vi "Example_Set_Get Functios.vi"() -> ()   [LabVIEW 2020]
doc: "Demonstrates the most used functions of the VI Server Toolkit - getting or setting control values based on two polymorphic VIs."
uses:
  VI Server Toolkit LV2013.lvlib
  VI Server Libraries/VI Server_Set Controls.llb/Set DBL SLIDE Control.vi
  VI Server Libraries/VI Server_Set Controls.llb/Set DBL Knob Control.vi
  VI Server Libraries/VI Server_Set Controls.llb/Set 1D STR Control.vi
  VI Server Libraries/VI Server_Set Controls.llb/Set STR Control.vi
panel:
  in  "Tab.Main":enum32{"Set/Get1", "Set/Get2"}(tab)
  in  "Menu Ring.Item Names":string[](array[string])=["Item 1", "Item 2", "Item 3"] caption="1D Array - String"
  in  "Slide.Get":bool
  in  "Slide.Set":bool
  in  "Menu Ring.Get":bool
  in  "Menu Ring.Set":bool
  in  "File Path.Source":path
  in  "Numeric.Source":dbl=5.0 caption="Numeric Control"
  in  "Slide.Source":dbl(slide)=1.9191919191919191 caption="Horizontal Fill Slide" scale=0.0..10.0
  in  "Knob.Source":dbl(knob)=1.6969989516945825 caption="Knob" scale=0.0..10.0
  in  "Button.Source":bool caption="Settings Button"
  in  "Menu Ring.Source":u16(ring) caption="Menu Ring" items=["Item 1", "Item 2", "Item 3"]
  in  "LED.Source":bool caption="LED"
  in  "File Path.Get":bool
  in  "File Path.Set":bool
  in  "LED.Get":bool
  in  "LED.Set":bool
  in  "Button.Get":bool
  in  "Button.Set":bool
  in  "Knob.Get":bool
  in  "Knob.Set":bool
  in  "Numeric.Get":bool
  in  "Numeric.Set":bool
  in  "File Path.Mirror":path
  in  "Numeric.Mirror":dbl=5.0 caption="Numeric Control"
  in  "Slide.Mirror":dbl(slide)=1.9191919191919191 caption="Horizontal Fill Slide" scale=0.0..10.0
  in  "Knob.Mirror":dbl(knob) caption="Knob" scale=0.0..10.0
  in  "Button.Mirror":bool caption="Settings Button"
  in  "Menu Ring.Mirror":u16(ring) caption="Menu Ring" items=["Item 1", "Item 2", "Item 3"]
  in  "LED.Mirror":bool caption="LED"
  in  "2D Array - Path.Get":bool
  in  "2D Array - Path.Set":bool
  in  "2D Array - DBL.Get":bool
  in  "2D Array - DBL.Set":bool
  in  "1D Array - DBL.Get":bool
  in  "1D Array - DBL.Set":bool
  in  "2D Array - String.Get":bool
  in  "2D Array - String.Set":bool
  in  "1D Array - String.Mirror":string[](array[string]) caption="1D Array - String"
  in  "2D Array - String.Mirror":string[][](array[string]) caption="2D Array - String"
  in  "1D Array - DBL.Mirror":dbl[](array[numeric]) caption="1D Array - DBL"
  in  "2D Array - DBL.Mirror":dbl[][](array[numeric]) caption="2D Array - DBL"
  in  "2D Array - Path.Mirror":path[][](array[path]) caption="2D Array - String"
  in  "2D Array - Boolean.Mirror":bool[][](array[boolean]) caption="2D Array - String"
  in  "1D Array - String.Source":string[](array[string]) caption="1D Array - String"
  in  "2D Array - String.Source":string[][](array[string])=[["", ""], ["", ""], ["", "qwe"]] caption="2D Array - String"
  in  "1D Array - DBL.Source":dbl[](array[numeric]) caption="1D Array - DBL"
  in  "2D Array - DBL.Source":dbl[][](array[numeric]) caption="2D Array - DBL"
  in  "2D Array - Path.Source":path[][](array[path]) caption="2D Array - String"
  in  "2D Array - Boolean.Source":bool[][](array[boolean]) caption="2D Array - String"
  in  "1D Array - String.Get":bool
  in  "1D Array - String.Set":bool
  in  "2D Array - Path.Get":bool
  in  "2D Array - Path.Set":bool
  in  "EXIT":bool=TRUE
  in  "Error In":errorcluster
  out "error out":errorcluster
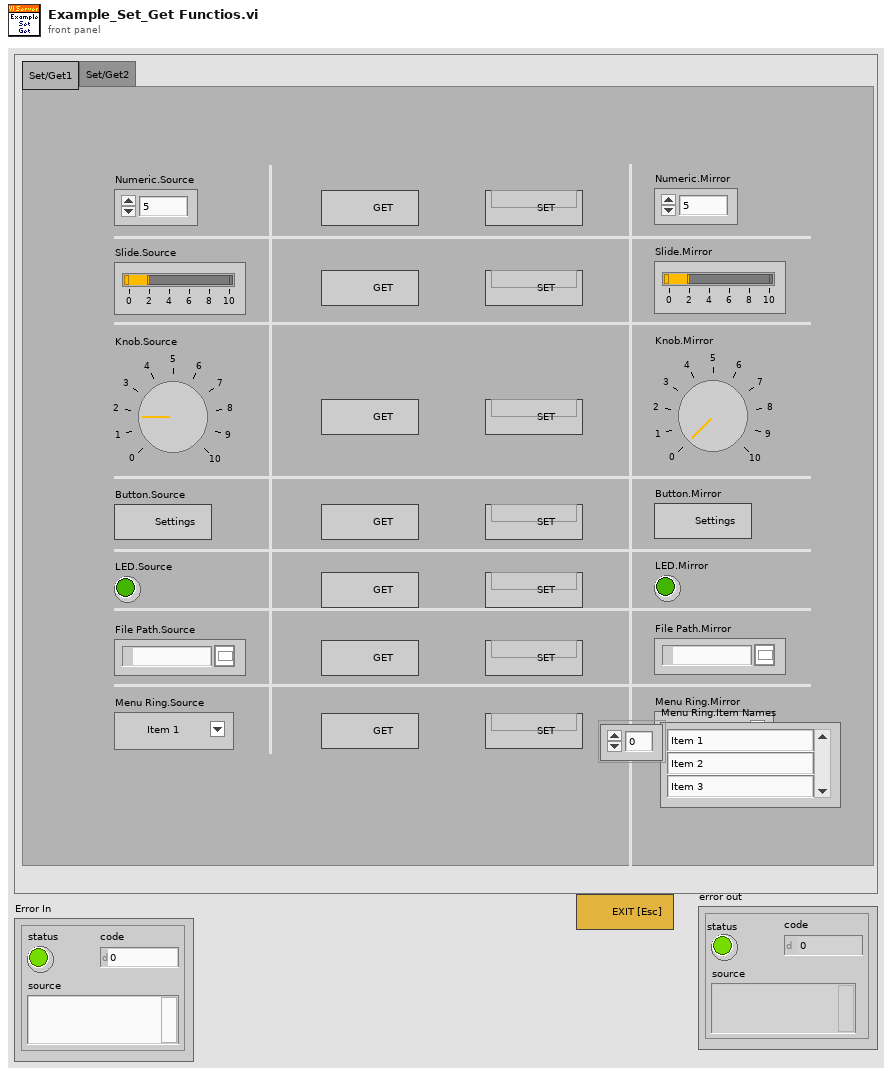
[diagram p1: front panel]
types:
  T1 = typedef "VI Server_RefsCluster.ctl" = cluster{"Labels":string[], "Refs":refnum<vi>[], "VI Ref":refnum<vi>}
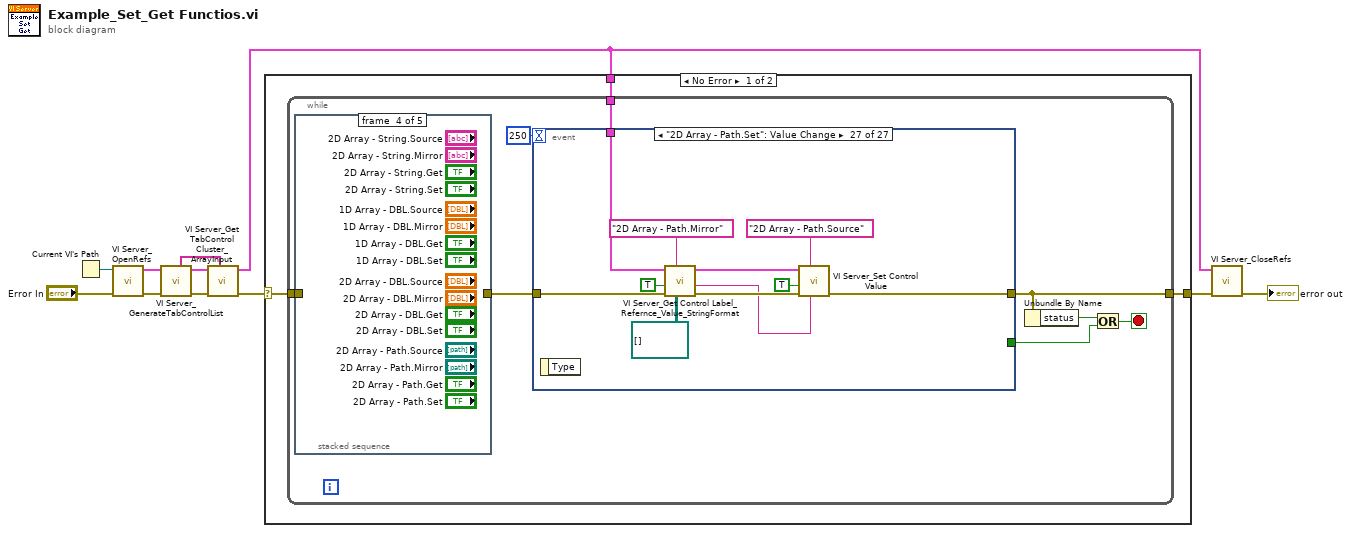
[diagram p0: block diagram]
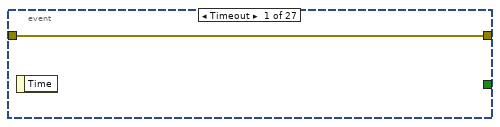
[diagram p2: hidden frame]
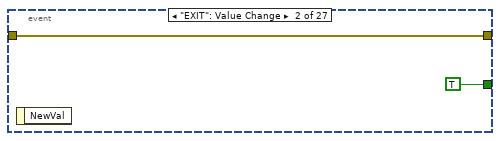
[diagram p3: hidden frame]
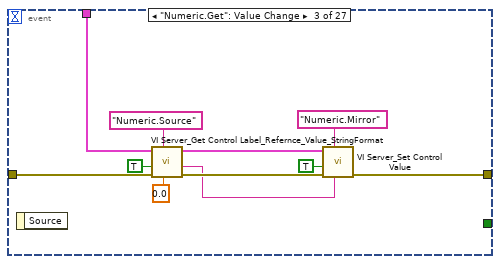
[diagram p4: hidden frame]
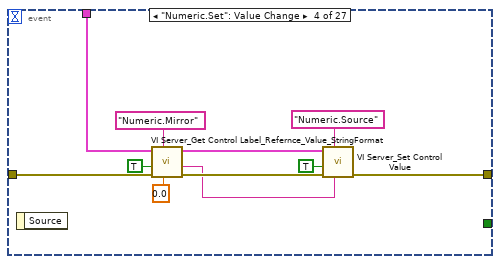
[diagram p5: hidden frame]
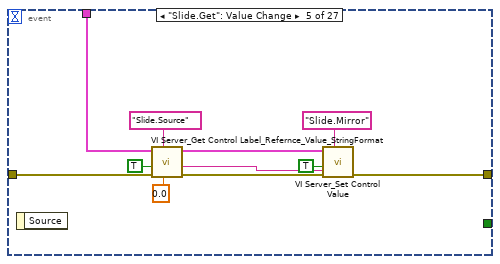
[diagram p6: hidden frame]
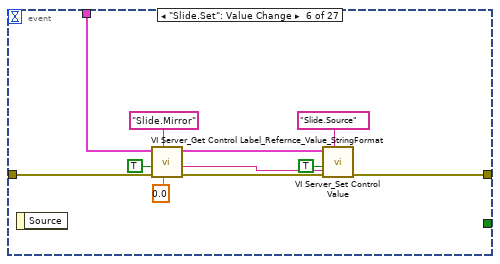
[diagram p7: hidden frame]
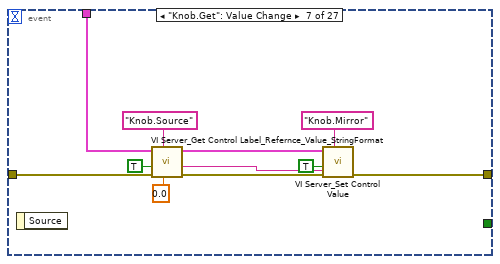
[diagram p8: hidden frame]
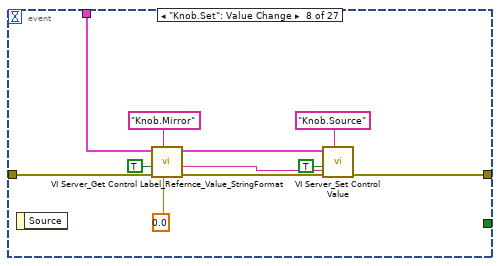
[diagram p9: hidden frame]
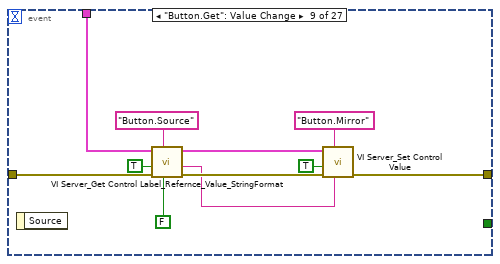
[diagram p10: hidden frame]
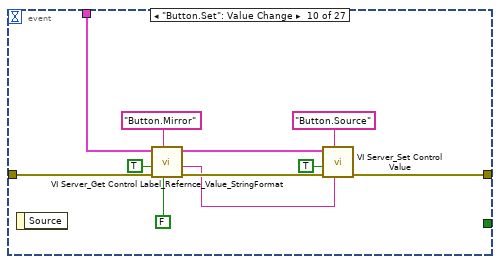
[diagram p11: hidden frame]
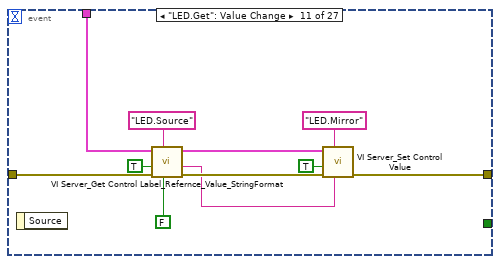
[diagram p12: hidden frame]
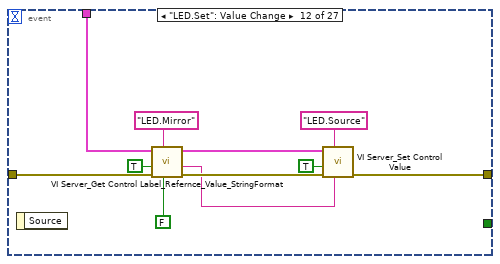
[diagram p13: hidden frame]
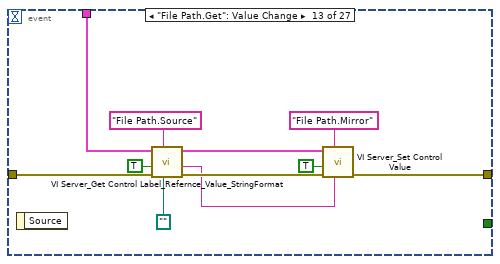
[diagram p14: hidden frame]
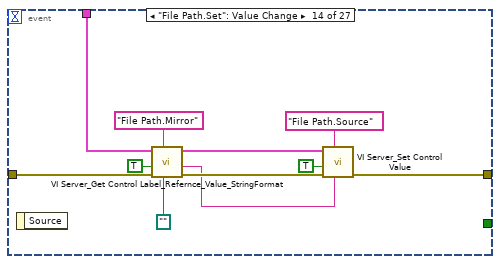
[diagram p15: hidden frame]
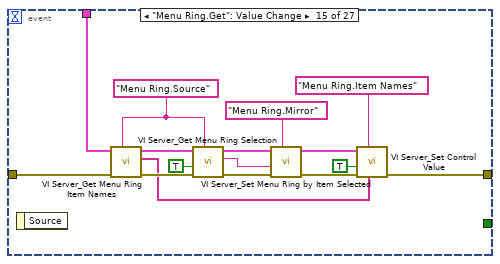
[diagram p16: hidden frame]
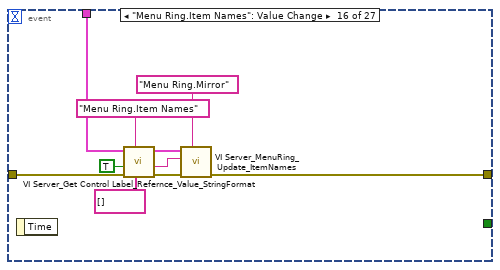
[diagram p17: hidden frame]
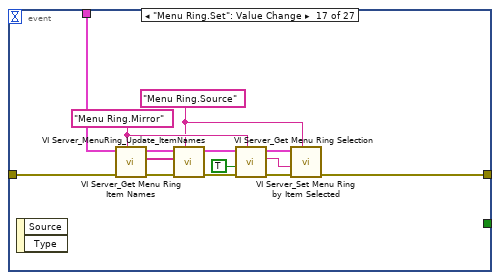
[diagram p18: hidden frame]
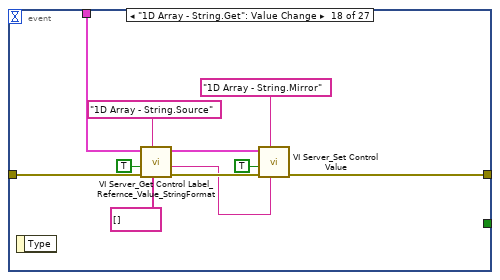
[diagram p19: hidden frame]
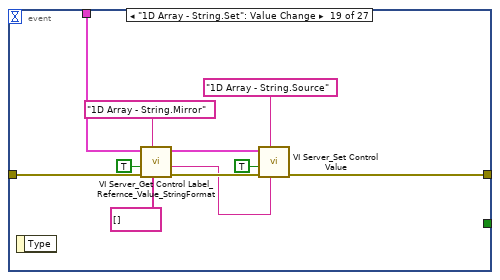
[diagram p20: hidden frame]
diagram:
  n1 = Current VI's Path() -> (path=w10:path)
  n2 = call "VI Server_OpenRefs.vi"("error in"="Error In", "VI Path"=w10) -> ("error out"=w4:errorcluster, "VI Server.RefsCluster"=w5:T1)  [unwired: 8 in]
  n3 = call "VI Server_GenerateTabControlList.vi"("error in (no error)"=w4, "VI Server Cluster"=w5) -> ("error out"=w7:errorcluster, "VI Server Cluster.DUP"=w6:T1, "TabControls"=w2:string[])  [unwired: 7 in]
  n4 = call "VI Server_Get TabControl Cluster_ArrayInput.vi"("TabControl Labels[]"=w2, "error in"=w7, "VI Server Cluster"=w6) -> ("error out"=w3:errorcluster, "VI Server Cluster.OUT"=w1:T1)  [unwired: 7 in]
  n5 = case shown="No Error" w3 {
    selector: w3 -> [w14 w309]
    tunnel: [w13 w309] -> w9
    tunnel: w1 -> [w12 _]
    frame No Error {
      n6 = while {
        tunnel: w14 -> [w21]
        tunnel: [w19] -> w13
        tunnel: w12 -> [w15]
        stop <- w16 stop-if-true
        n7 = stacked-sequence {
          tunnel: [w308 _ _ _ _] -> w20
          tunnel: w21 -> [w308 _ _ _ _]
          frame #0 {
          }
          frame #1 {
          }
          frame #2 {
          }
          frame #3 {
          }
          frame #4 {
          }
        }
        n8 = event shown="[26] \"2D Array - Path.Set\": Value Change" {
          selector: _ -> [_ _ _ _ _ _ _ _ _ _ _ _ _ _ _ _ _ _ _ _ _ _ _ _ _ _ _]
          dyn-events: _ -> [_ _ _ _ _ _ _ _ _ _ _ _ _ _ _ _ _ _ _ _ _ _ _ _ _ _ _]
          timeout: 250 -> [_ _ _ _ _ _ _ _ _ _ _ _ _ _ _ _ _ _ _ _ _ _ _ _ _ _ _]
          tunnel: w20 -> [w23 w25 w36 w47 w58 w69 w80 w91 w102 w113 w124 w135 w146 w157 w165 w183 w197 w208 w219 w230 w241 w252 w263 w274 w285 w296 w307]
          tunnel: [w23 w25 w30 w41 w52 w63 w74 w85 w96 w107 w118 w129 w140 w151 w159 w174 w186 w200 w211 w222 w233 w244 w255 w266 w277 w288 w299] -> w19
          tunnel: [_ TRUE _ _ _ _ _ _ _ _ _ _ _ _ _ _ _ _ _ _ _ _ _ _ _ _ _] -> w17
          tunnel: w15 -> [_ _ w35 w46 w57 w68 w79 w90 w101 w112 w123 w134 w145 w156 w163 w182 w196 w207 w218 w229 w240 w251 w262 w273 w284 w295 w306]
          event Timeout {
            n9 = event-data() -> ()  [unwired: 1 in, 1 out]
          }
          event "EXIT": Value Change {
            n10 = event-data() -> ()  [unwired: 1 in, 1 out]
          }
          event "Numeric.Get": Value Change {
            n11 = event-data() -> ()  [unwired: 1 in, 1 out]
            n12 = call "VI Server_Get Control Label_Refernce_Value_StringFormat.vi"(6:0.0, "Label"="Numeric.Source", "error in (no error)"=w36, 9:TRUE ("Single Instance (T)"), "VI Server Cluster"=w35) -> ("error out"=w31:errorcluster, "ControlValue(StringFormat)"=w27:string, "VI Server Cluster.DUP"=w28:T1)  [unwired: 4 in]
            n13 = call-poly "VI Server_Set Control Value.vi"("New Value"=w27, "Label"="Numeric.Mirror", "error in"=w31, "Single Instance (T)"=TRUE, "VI Server Cluster"=w28) -> ("error out"=w30:errorcluster)  [unwired: 4 in, 2 out]
          }
          event "Numeric.Set": Value Change {
            n14 = event-data() -> ()  [unwired: 1 in, 1 out]
            n15 = call "VI Server_Get Control Label_Refernce_Value_StringFormat.vi"(6:0.0, "Label"="Numeric.Mirror", "error in (no error)"=w47, 9:TRUE ("Single Instance (T)"), "VI Server Cluster"=w46) -> ("error out"=w42:errorcluster, "ControlValue(StringFormat)"=w38:string, "VI Server Cluster.DUP"=w39:T1)  [unwired: 4 in]
            n16 = call-poly "VI Server_Set Control Value.vi"("New Value"=w38, "Label"="Numeric.Source", "error in"=w42, "Single Instance (T)"=TRUE, "VI Server Cluster"=w39) -> ("error out"=w41:errorcluster)  [unwired: 4 in, 2 out]
          }
          event "Slide.Get": Value Change {
            n17 = event-data() -> ()  [unwired: 1 in, 1 out]
            n18 = call "VI Server_Get Control Label_Refernce_Value_StringFormat.vi"(6:0.0, "Label"="Slide.Source", "error in (no error)"=w58, 9:TRUE ("Single Instance (T)"), "VI Server Cluster"=w57) -> ("error out"=w53:errorcluster, "ControlValue(StringFormat)"=w49:string, "VI Server Cluster.DUP"=w50:T1)  [unwired: 4 in]
            n19 = call-poly "VI Server_Set Control Value.vi"("New Value"=w49, "Label"="Slide.Mirror", "error in"=w53, "Single Instance (T)"=TRUE, "VI Server Cluster"=w50) -> ("error out"=w52:errorcluster)  [unwired: 4 in, 2 out]
          }
          event "Slide.Set": Value Change {
            n20 = event-data() -> ()  [unwired: 1 in, 1 out]
            n21 = call "VI Server_Get Control Label_Refernce_Value_StringFormat.vi"(6:0.0, "Label"="Slide.Mirror", "error in (no error)"=w69, 9:TRUE ("Single Instance (T)"), "VI Server Cluster"=w68) -> ("error out"=w64:errorcluster, "ControlValue(StringFormat)"=w60:string, "VI Server Cluster.DUP"=w61:T1)  [unwired: 4 in]
            n22 = call-poly "VI Server_Set Control Value.vi"("New Value"=w60, "Label"="Slide.Source", "error in"=w64, "Single Instance (T)"=TRUE, "VI Server Cluster"=w61) -> ("error out"=w63:errorcluster)  [unwired: 4 in, 2 out]
          }
          event "Knob.Get": Value Change {
            n23 = event-data() -> ()  [unwired: 1 in, 1 out]
            n24 = call "VI Server_Get Control Label_Refernce_Value_StringFormat.vi"(6:0.0, "Label"="Knob.Source", "error in (no error)"=w80, 9:TRUE ("Single Instance (T)"), "VI Server Cluster"=w79) -> ("error out"=w75:errorcluster, "ControlValue(StringFormat)"=w71:string, "VI Server Cluster.DUP"=w72:T1)  [unwired: 4 in]
            n25 = call-poly "VI Server_Set Control Value.vi"("New Value"=w71, "Label"="Knob.Mirror", "error in"=w75, "Single Instance (T)"=TRUE, "VI Server Cluster"=w72) -> ("error out"=w74:errorcluster)  [unwired: 4 in, 2 out]
          }
          event "Knob.Set": Value Change {
            n26 = event-data() -> ()  [unwired: 1 in, 1 out]
            n27 = call "VI Server_Get Control Label_Refernce_Value_StringFormat.vi"(6:0.0, "Label"="Knob.Mirror", "error in (no error)"=w91, 9:TRUE ("Single Instance (T)"), "VI Server Cluster"=w90) -> ("error out"=w86:errorcluster, "ControlValue(StringFormat)"=w82:string, "VI Server Cluster.DUP"=w83:T1)  [unwired: 4 in]
            n28 = call-poly "VI Server_Set Control Value.vi"("New Value"=w82, "Label"="Knob.Source", "error in"=w86, "Single Instance (T)"=TRUE, "VI Server Cluster"=w83) -> ("error out"=w85:errorcluster)  [unwired: 4 in, 2 out]
          }
          event "Button.Get": Value Change {
            n29 = event-data() -> ()  [unwired: 1 in, 1 out]
            n30 = call "VI Server_Get Control Label_Refernce_Value_StringFormat.vi"(6:FALSE, "Label"="Button.Source", "error in (no error)"=w102, 9:TRUE ("Single Instance (T)"), "VI Server Cluster"=w101) -> ("error out"=w97:errorcluster, "ControlValue(StringFormat)"=w93:string, "VI Server Cluster.DUP"=w94:T1)  [unwired: 4 in]
            n31 = call-poly "VI Server_Set Control Value.vi"("New Value"=w93, "Label"="Button.Mirror", "error in"=w97, "Single Instance (T)"=TRUE, "VI Server Cluster"=w94) -> ("error out"=w96:errorcluster)  [unwired: 4 in, 2 out]
          }
          event "Button.Set": Value Change {
            n32 = event-data() -> ()  [unwired: 1 in, 1 out]
            n33 = call "VI Server_Get Control Label_Refernce_Value_StringFormat.vi"(6:FALSE, "Label"="Button.Mirror", "error in (no error)"=w113, 9:TRUE ("Single Instance (T)"), "VI Server Cluster"=w112) -> ("error out"=w108:errorcluster, "ControlValue(StringFormat)"=w104:string, "VI Server Cluster.DUP"=w105:T1)  [unwired: 4 in]
            n34 = call-poly "VI Server_Set Control Value.vi"("New Value"=w104, "Label"="Button.Source", "error in"=w108, "Single Instance (T)"=TRUE, "VI Server Cluster"=w105) -> ("error out"=w107:errorcluster)  [unwired: 4 in, 2 out]
          }
          event "LED.Get": Value Change {
            n35 = event-data() -> ()  [unwired: 1 in, 1 out]
            n36 = call "VI Server_Get Control Label_Refernce_Value_StringFormat.vi"(6:FALSE, "Label"="LED.Source", "error in (no error)"=w124, 9:TRUE ("Single Instance (T)"), "VI Server Cluster"=w123) -> ("error out"=w119:errorcluster, "ControlValue(StringFormat)"=w115:string, "VI Server Cluster.DUP"=w116:T1)  [unwired: 4 in]
            n37 = call-poly "VI Server_Set Control Value.vi"("New Value"=w115, "Label"="LED.Mirror", "error in"=w119, "Single Instance (T)"=TRUE, "VI Server Cluster"=w116) -> ("error out"=w118:errorcluster)  [unwired: 4 in, 2 out]
          }
          event "LED.Set": Value Change {
            n38 = event-data() -> ()  [unwired: 1 in, 1 out]
            n39 = call "VI Server_Get Control Label_Refernce_Value_StringFormat.vi"(6:FALSE, "Label"="LED.Mirror", "error in (no error)"=w135, 9:TRUE ("Single Instance (T)"), "VI Server Cluster"=w134) -> ("error out"=w130:errorcluster, "ControlValue(StringFormat)"=w126:string, "VI Server Cluster.DUP"=w127:T1)  [unwired: 4 in]
            n40 = call-poly "VI Server_Set Control Value.vi"("New Value"=w126, "Label"="LED.Source", "error in"=w130, "Single Instance (T)"=TRUE, "VI Server Cluster"=w127) -> ("error out"=w129:errorcluster)  [unwired: 4 in, 2 out]
          }
          event "File Path.Get": Value Change {
            n41 = event-data() -> ()  [unwired: 1 in, 1 out]
            n42 = call "VI Server_Get Control Label_Refernce_Value_StringFormat.vi"(6:path "", "Label"="File Path.Source", "error in (no error)"=w146, 9:TRUE ("Single Instance (T)"), "VI Server Cluster"=w145) -> ("error out"=w141:errorcluster, "ControlValue(StringFormat)"=w137:string, "VI Server Cluster.DUP"=w138:T1)  [unwired: 4 in]
            n43 = call-poly "VI Server_Set Control Value.vi"("New Value"=w137, "Label"="File Path.Mirror", "error in"=w141, "Single Instance (T)"=TRUE, "VI Server Cluster"=w138) -> ("error out"=w140:errorcluster)  [unwired: 4 in, 2 out]
          }
          event "File Path.Set": Value Change {
            n44 = event-data() -> ()  [unwired: 1 in, 1 out]
            n45 = call "VI Server_Get Control Label_Refernce_Value_StringFormat.vi"(6:path "", "Label"="File Path.Mirror", "error in (no error)"=w157, 9:TRUE ("Single Instance (T)"), "VI Server Cluster"=w156) -> ("error out"=w152:errorcluster, "ControlValue(StringFormat)"=w148:string, "VI Server Cluster.DUP"=w149:T1)  [unwired: 4 in]
            n46 = call-poly "VI Server_Set Control Value.vi"("New Value"=w148, "Label"="File Path.Source", "error in"=w152, "Single Instance (T)"=TRUE, "VI Server Cluster"=w149) -> ("error out"=w151:errorcluster)  [unwired: 4 in, 2 out]
          }
          event "Menu Ring.Get": Value Change {
            w161 = "Menu Ring.Source" ("Label")
            n47 = event-data() -> ()  [unwired: 1 in, 1 out]
            n48 = call "VI Server_Get Menu Ring Item Names.vi"("Label"=w161, "error in"=w165, "VI Server Cluster"=w163) -> ("error out"=w164:errorcluster, "Item Names (String[])"=w160:string[], "VI Server Cluster.DUP"=w162:T1)  [unwired: 3 in, 3 out]
            n49 = call "VI Server_Get Menu Ring Selection.vi"("Label"=w161, "error in"=w164, "Single Instance (T)"=TRUE, "VI Server Cluster"=w162) -> ("error out"=w172:errorcluster, "Selection"=w170:string, "VI Server Cluster.DUP"=w167:T1)  [unwired: 2 in, 3 out]
            n50 = call "VI Server_Set Menu Ring by Item Selected.vi"("Label"="Menu Ring.Mirror", "error in"=w172, "Item"=w170, "VI Server Cluster"=w167) -> ("error out"=w169:errorcluster, "VI Server Cluster.DUP"=w168:T1)  [unwired: 5 in, 1 out]
            n51 = call-poly "VI Server_Set Control Value.vi"("New Value"=w160, "Label"="Menu Ring.Item Names", "error in"=w169, "Single Instance (T)"=TRUE, "VI Server Cluster"=w168) -> ("error out"=w159:errorcluster)  [unwired: 4 in, 2 out]
          }
          event "Menu Ring.Item Names": Value Change {
            n52 = event-data() -> ()  [unwired: 1 in, 1 out]
            n53 = call "VI Server_Get Control Label_Refernce_Value_StringFormat.vi"(6:string[] [], "Label"="Menu Ring.Item Names", "error in (no error)"=w183, 9:TRUE ("Single Instance (T)"), "VI Server Cluster"=w182) -> ("error out"=w178:errorcluster, "ControlValue(StringFormat)"=w175:string, "VI Server Cluster.DUP"=w177:T1)  [unwired: 4 in]
            n54 = call "VI Server_MenuRing_Update_ItemNames.vi"("Label"="Menu Ring.Mirror", "error in"=w178, "Strings []"=w175, "VI Server Cluster"=w177) -> ("error out"=w174:errorcluster)  [unwired: 5 in, 2 out]
          }
          event "Menu Ring.Set": Value Change {
            w185 = "Menu Ring.Source"
            w191 = "Menu Ring.Mirror"
            n55 = event-data() -> ()  [unwired: 1 in, 2 out]
            n56 = call "VI Server_Get Menu Ring Item Names.vi"("Label"=w191, "error in"=w197, "VI Server Cluster"=w196) -> ("error out"=w195:errorcluster, "Item Names (String[])"=w193:string[], "VI Server Cluster.DUP"=w194:T1)  [unwired: 3 in, 3 out]
            n57 = call "VI Server_MenuRing_Update_ItemNames.vi"("Label"=w185, "error in"=w195, "Strings []"=w193, "VI Server Cluster"=w194) -> ("error out"=w192:errorcluster, "VI Server Cluster.DUP"=w190:T1)  [unwired: 5 in, 1 out]
            n58 = call "VI Server_Get Menu Ring Selection.vi"("Label"=w191, "error in"=w192, "Single Instance (T)"=TRUE, "VI Server Cluster"=w190) -> ("error out"=w188:errorcluster, "Selection"=w184:string, "VI Server Cluster.DUP"=w187:T1)  [unwired: 2 in, 3 out]
            n59 = call "VI Server_Set Menu Ring by Item Selected.vi"("Label"=w185, "error in"=w188, "Item"=w184, "VI Server Cluster"=w187) -> ("error out"=w186:errorcluster)  [unwired: 5 in, 2 out]
          }
          event "1D Array - String.Get": Value Change {
            n60 = event-data() -> ()  [unwired: 1 in, 1 out]
            n61 = call "VI Server_Get Control Label_Refernce_Value_StringFormat.vi"(6:string[] [], "Label"="1D Array - String.Source", "error in (no error)"=w208, 9:TRUE ("Single Instance (T)"), "VI Server Cluster"=w207) -> ("error out"=w203:errorcluster, "ControlValue(StringFormat)"=w198:string, "VI Server Cluster.DUP"=w202:T1)  [unwired: 4 in]
            n62 = call-poly "VI Server_Set Control Value.vi"("New Value"=w198, "Label"="1D Array - String.Mirror", "error in"=w203, "Single Instance (T)"=TRUE, "VI Server Cluster"=w202) -> ("error out"=w200:errorcluster)  [unwired: 4 in, 2 out]
          }
          event "1D Array - String.Set": Value Change {
            n63 = event-data() -> ()  [unwired: 1 in, 1 out]
            n64 = call "VI Server_Get Control Label_Refernce_Value_StringFormat.vi"(6:string[] [], "Label"="1D Array - String.Mirror", "error in (no error)"=w219, 9:TRUE ("Single Instance (T)"), "VI Server Cluster"=w218) -> ("error out"=w214:errorcluster, "ControlValue(StringFormat)"=w209:string, "VI Server Cluster.DUP"=w213:T1)  [unwired: 4 in]
            n65 = call-poly "VI Server_Set Control Value.vi"("New Value"=w209, "Label"="1D Array - String.Source", "error in"=w214, "Single Instance (T)"=TRUE, "VI Server Cluster"=w213) -> ("error out"=w211:errorcluster)  [unwired: 4 in, 2 out]
          }
          event "2D Array - String.Get": Value Change {
            n66 = event-data() -> ()  [unwired: 1 in, 1 out]
            n67 = call "VI Server_Get Control Label_Refernce_Value_StringFormat.vi"(6:string[][] [], "Label"="2D Array - String.Source", "error in (no error)"=w230, 9:TRUE ("Single Instance (T)"), "VI Server Cluster"=w229) -> ("error out"=w225:errorcluster, "ControlValue(StringFormat)"=w220:string, "VI Server Cluster.DUP"=w224:T1)  [unwired: 4 in]
            n68 = call-poly "VI Server_Set Control Value.vi"("New Value"=w220, "Label"="2D Array - String.Mirror", "error in"=w225, "Single Instance (T)"=TRUE, "VI Server Cluster"=w224) -> ("error out"=w222:errorcluster)  [unwired: 4 in, 2 out]
          }
          event "2D Array - String.Set": Value Change {
            n69 = event-data() -> ()  [unwired: 1 in, 1 out]
            n70 = call "VI Server_Get Control Label_Refernce_Value_StringFormat.vi"(6:string[][] [], "Label"="2D Array - String.Mirror", "error in (no error)"=w241, 9:TRUE ("Single Instance (T)"), "VI Server Cluster"=w240) -> ("error out"=w236:errorcluster, "ControlValue(StringFormat)"=w231:string, "VI Server Cluster.DUP"=w235:T1)  [unwired: 4 in]
            n71 = call-poly "VI Server_Set Control Value.vi"("New Value"=w231, "Label"="2D Array - String.Source", "error in"=w236, "Single Instance (T)"=TRUE, "VI Server Cluster"=w235) -> ("error out"=w233:errorcluster)  [unwired: 4 in, 2 out]
          }
          event "1D Array - DBL.Get": Value Change {
            n72 = event-data() -> ()  [unwired: 1 in, 1 out]
            n73 = call "VI Server_Get Control Label_Refernce_Value_StringFormat.vi"(6:dbl[] [], "Label"="1D Array - DBL.Source", "error in (no error)"=w252, 9:TRUE ("Single Instance (T)"), "VI Server Cluster"=w251) -> ("error out"=w247:errorcluster, "ControlValue(StringFormat)"=w242:string, "VI Server Cluster.DUP"=w246:T1)  [unwired: 4 in]
            n74 = call-poly "VI Server_Set Control Value.vi"("New Value"=w242, "Label"="1D Array - DBL.Mirror", "error in"=w247, "Single Instance (T)"=TRUE, "VI Server Cluster"=w246) -> ("error out"=w244:errorcluster)  [unwired: 4 in, 2 out]
          }
          event "1D Array - DBL.Set": Value Change {
            n75 = event-data() -> ()  [unwired: 1 in, 1 out]
            n76 = call "VI Server_Get Control Label_Refernce_Value_StringFormat.vi"(6:dbl[] [], "Label"="1D Array - DBL.Mirror", "error in (no error)"=w263, 9:TRUE ("Single Instance (T)"), "VI Server Cluster"=w262) -> ("error out"=w258:errorcluster, "ControlValue(StringFormat)"=w253:string, "VI Server Cluster.DUP"=w257:T1)  [unwired: 4 in]
            n77 = call-poly "VI Server_Set Control Value.vi"("New Value"=w253, "Label"="1D Array - DBL.Source", "error in"=w258, "Single Instance (T)"=TRUE, "VI Server Cluster"=w257) -> ("error out"=w255:errorcluster)  [unwired: 4 in, 2 out]
          }
          event "2D Array - DBL.Get": Value Change {
            n78 = event-data() -> ()  [unwired: 1 in, 1 out]
            n79 = call "VI Server_Get Control Label_Refernce_Value_StringFormat.vi"(6:dbl[][] [], "Label"="2D Array - DBL.Source", "error in (no error)"=w274, 9:TRUE ("Single Instance (T)"), "VI Server Cluster"=w273) -> ("error out"=w269:errorcluster, "ControlValue(StringFormat)"=w264:string, "VI Server Cluster.DUP"=w268:T1)  [unwired: 4 in]
            n80 = call-poly "VI Server_Set Control Value.vi"("New Value"=w264, "Label"="2D Array - DBL.Mirror", "error in"=w269, "Single Instance (T)"=TRUE, "VI Server Cluster"=w268) -> ("error out"=w266:errorcluster)  [unwired: 4 in, 2 out]
          }
          event "2D Array - DBL.Set": Value Change {
            n81 = event-data() -> ()  [unwired: 1 in, 1 out]
            n82 = call "VI Server_Get Control Label_Refernce_Value_StringFormat.vi"(6:dbl[][] [], "Label"="2D Array - DBL.Mirror", "error in (no error)"=w285, 9:TRUE ("Single Instance (T)"), "VI Server Cluster"=w284) -> ("error out"=w280:errorcluster, "ControlValue(StringFormat)"=w275:string, "VI Server Cluster.DUP"=w279:T1)  [unwired: 4 in]
            n83 = call-poly "VI Server_Set Control Value.vi"("New Value"=w275, "Label"="2D Array - DBL.Source", "error in"=w280, "Single Instance (T)"=TRUE, "VI Server Cluster"=w279) -> ("error out"=w277:errorcluster)  [unwired: 4 in, 2 out]
          }
          event "2D Array - Path.Get": Value Change {
            n84 = event-data() -> ()  [unwired: 1 in, 1 out]
            n85 = call "VI Server_Get Control Label_Refernce_Value_StringFormat.vi"(6:path[][] [], "Label"="2D Array - Path.Source", "error in (no error)"=w296, 9:TRUE ("Single Instance (T)"), "VI Server Cluster"=w295) -> ("error out"=w291:errorcluster, "ControlValue(StringFormat)"=w286:string, "VI Server Cluster.DUP"=w290:T1)  [unwired: 4 in]
            n86 = call-poly "VI Server_Set Control Value.vi"("New Value"=w286, "Label"="2D Array - Path.Mirror", "error in"=w291, "Single Instance (T)"=TRUE, "VI Server Cluster"=w290) -> ("error out"=w288:errorcluster)  [unwired: 4 in, 2 out]
          }
          event "2D Array - Path.Set": Value Change {
            n87 = event-data() -> ()  [unwired: 1 in, 1 out]
            n88 = call "VI Server_Get Control Label_Refernce_Value_StringFormat.vi"(6:path[][] [], "Label"="2D Array - Path.Mirror", "error in (no error)"=w307, 9:TRUE ("Single Instance (T)"), "VI Server Cluster"=w306) -> ("error out"=w302:errorcluster, "ControlValue(StringFormat)"=w297:string, "VI Server Cluster.DUP"=w301:T1)  [unwired: 4 in]
            n89 = call-poly "VI Server_Set Control Value.vi"("New Value"=w297, "Label"="2D Array - Path.Source", "error in"=w302, "Single Instance (T)"=TRUE, "VI Server Cluster"=w301) -> ("error out"=w299:errorcluster)  [unwired: 4 in, 2 out]
          }
        }
        n90 = Unbundle By Name(w19) -> ("status"=w18:bool)
        n91 = Or(x=w18, y=w17) -> (x .or. y?=w16:bool)
      }
    }
    frame Error {
    }
  }
  n92 = call "VI Server_CloseRefs.vi"("error in"=w9, "VI Server.RefsCluster"=w1) -> ("error out"=→"error out":errorcluster)  [unwired: 9 in]
